vi "WS Client Ready.vi"(8 "error in (no error)":errorcluster, 10 "WebSocket Client":refnum<class "WebSocket Client.lvclass">, 11 "WebSocket Manager in":refnum<class "WebSocket Manager.lvclass">) -> (0 "error out":errorcluster)   [LabVIEW 2020, in "HTTP Server.lvlib" / "WebSocket Manager.lvclass"]
uses:
  WebSocket Manager.lvclass
  WebSocket Client/WebSocket Client.lvclass
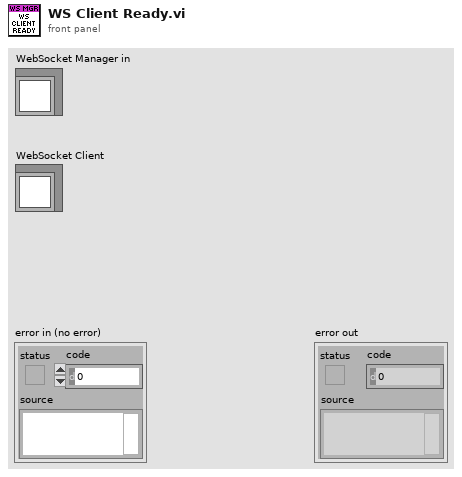
[diagram p1: front panel]
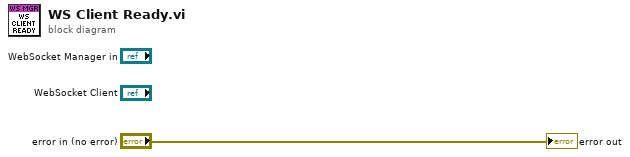
[diagram p0: block diagram]
diagram:
  "error out" <- "error in (no error)"
